vi "SubPanel.vi"(0 "DVR In":refnum<data-value>, 5 "Speed Mode":string, 11 "error in (no error)":errorcluster) -> (4 "DVR Out":refnum<data-value>, 15 "error out":errorcluster)   [LabVIEW 2020, in "Low Speed.lvclass"]
uses:
  Low Speed.lvclass
  Parent/TX Speed.lvclass
  TypeDef/Timing Parameters Cluster.ctl
  TypeDef/User LV2 Mode Select.ctl
  Parent/TypeDefs/TX_Mode Queue Operation Mode.ctl
  TypeDef/Queue Operation Mode.ctl
  <vilib>/Utility/config.llb/Read Key (U32).vi
  I2C Controller Lib.lvlib
  <vilib>/Utility/config.llb/NI_LVConfig.lvlib
panel:
  in  "Time Params":T1={"f_SCL(KHz)"=100, "t_HIGH (ns)"=5000, "t_LOW (ns)"=5000, "t_SU;STA (ns)"=4700, "t_HD;STA (ns)"=4000, "t_SU;DAT (ns)"=2500, "t_HD;DAT (ns)"=2500, "t_SU;STO (ns)"=4000, "t_BUF (ns)"=4700} caption="Time Parameters" {"t_HIGH (ns)" max=1000000 step=1 format="%#.0f"; "t_LOW (ns)" max=1000000 step=1 format="%#.0f"; "f_SCL(KHz)" min=10 max=1000 step=1}
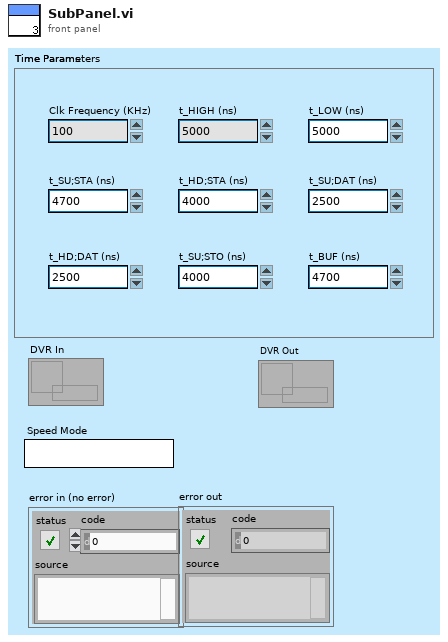
[diagram p1: front panel]
types:
  T1 = typedef "I2C Controller Lib.lvlib/Timing Parameters Cluster.ctl" = cluster{"f_SCL(KHz)":u32, "t_HIGH (ns)":u32, "t_LOW (ns)":u32, "t_SU;STA (ns)":u32, "t_HD;STA (ns)":u32, "t_SU;DAT (ns)":u32, "t_HD;DAT (ns)":u32, "t_SU;STO (ns)":u32, "t_BUF (ns)":u32}
  T2 = cluster{"DVR":refnum<data-value>, "Speed Mode":string, "Time Params":T1, "Event Ref.":refnum<event-registration>}
  T3 = typedef "TX Speed.lvclass/TX_Mode Queue Operation Mode.ctl" = enum16{"Create Q", "Enqueue", "Enqueue N", "Enstack", "Dequeue", "Flush Q", "Close Q"}
  T4 = typedef "I2C Controller Lib.lvlib/User LV2 Mode Select.ctl" = enum16{"Create", "Delete", "Stop"}
  T5 = typedef "I2C Controller Lib.lvlib/Queue Operation Mode.ctl" = enum16{"Create Q", "Enqueue", "Enqueue N", "Enstack", "Dequeue", "Flush Q", "Close Q"}
  T6 = typedef "NI_LVConfig.lvlib/Config Data RefNum.ctl" = refnum<k1>
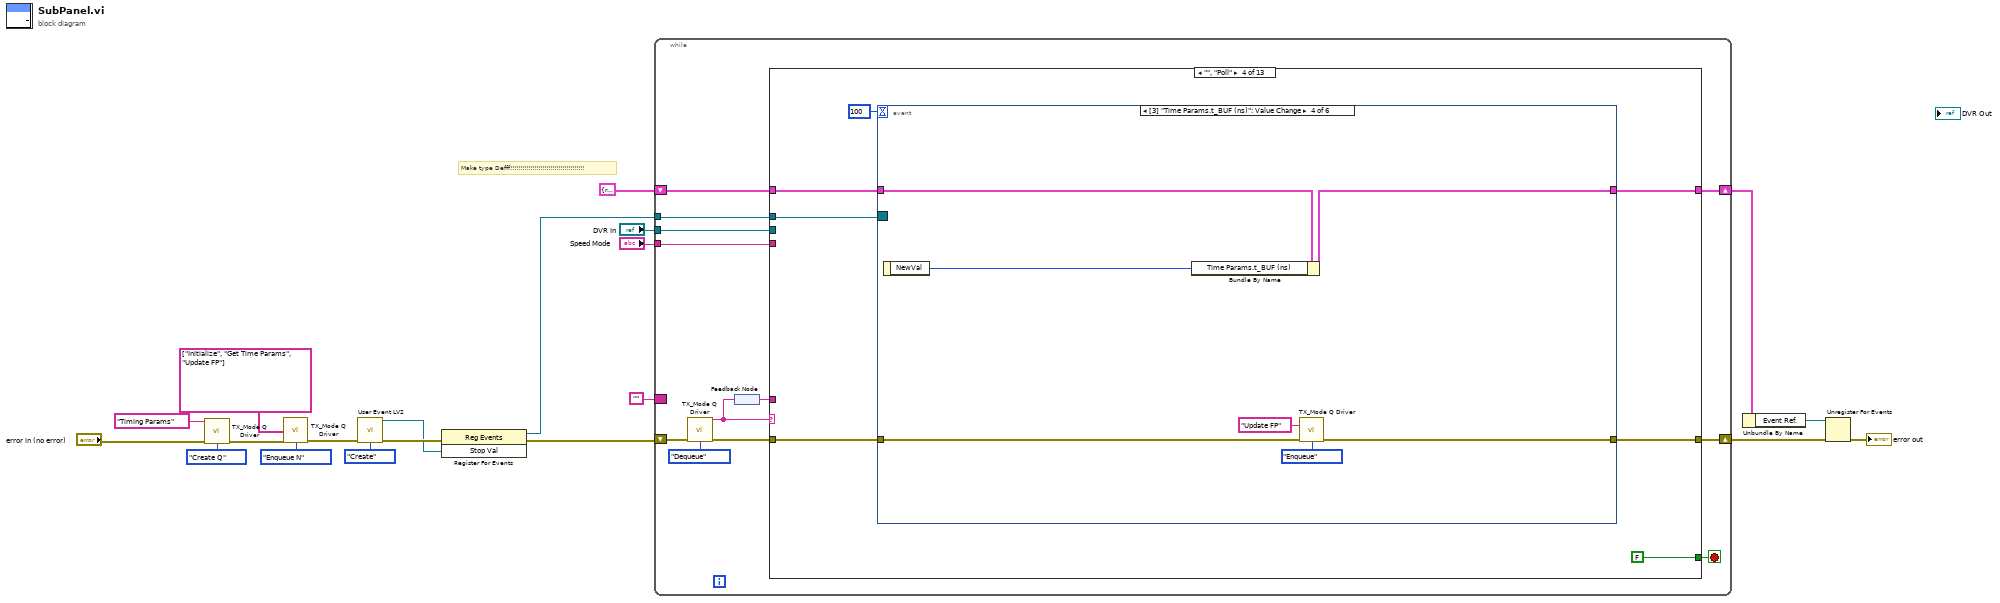
[diagram p0: block diagram]
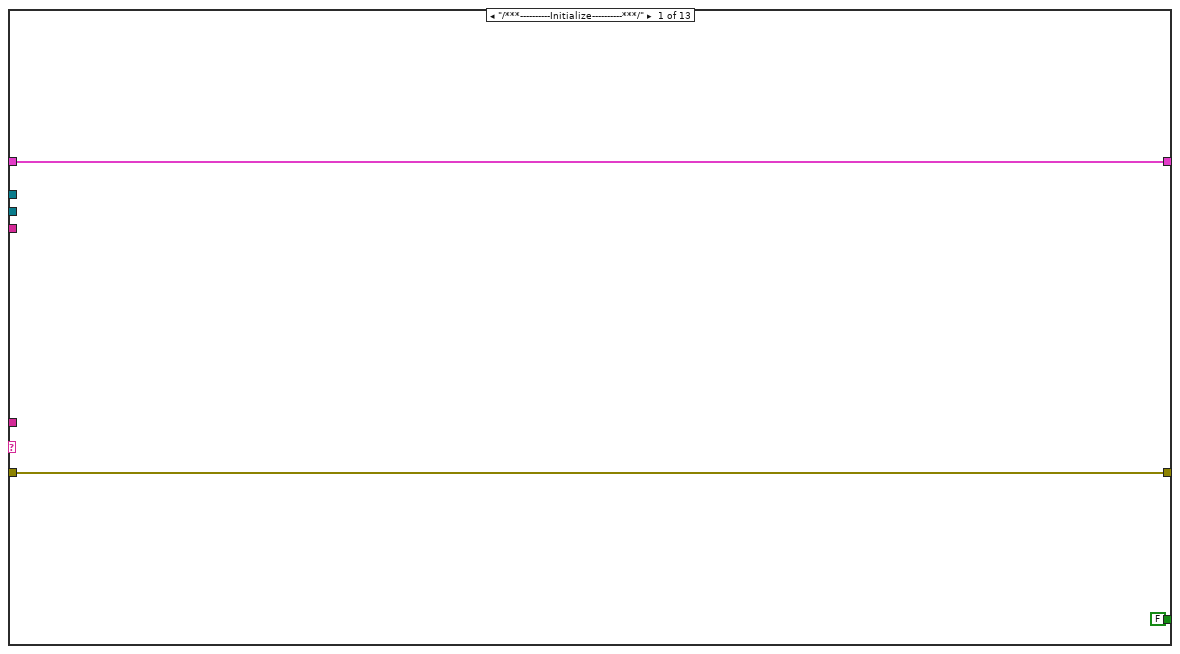
[diagram p2: hidden frame]
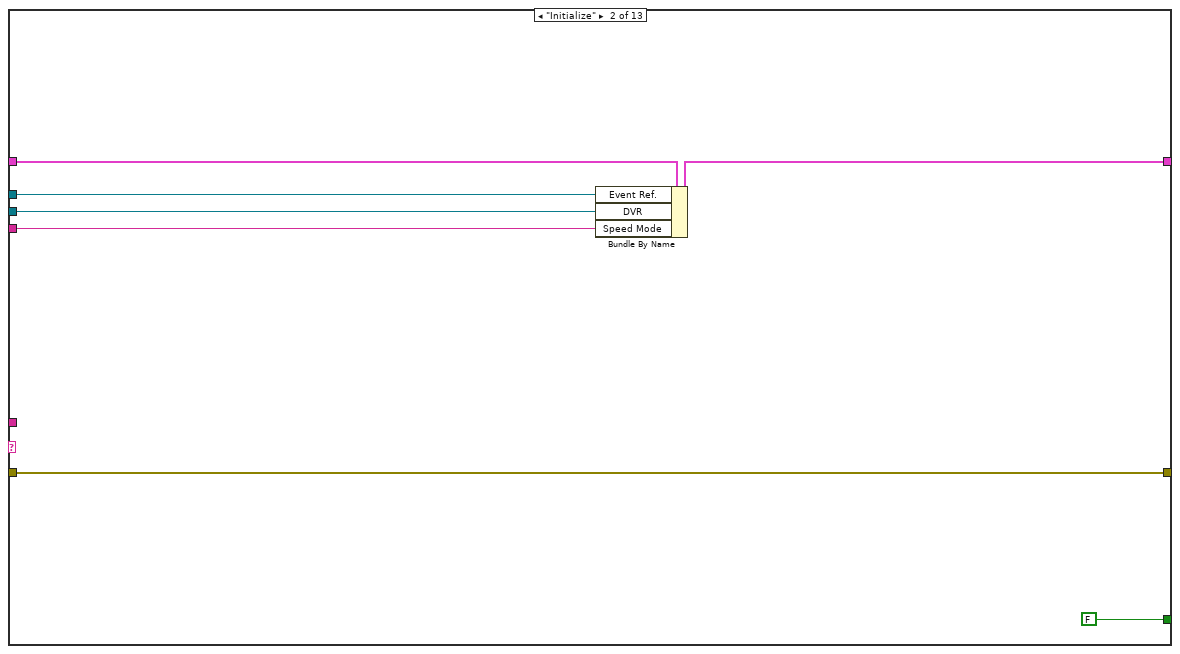
[diagram p3: hidden frame]
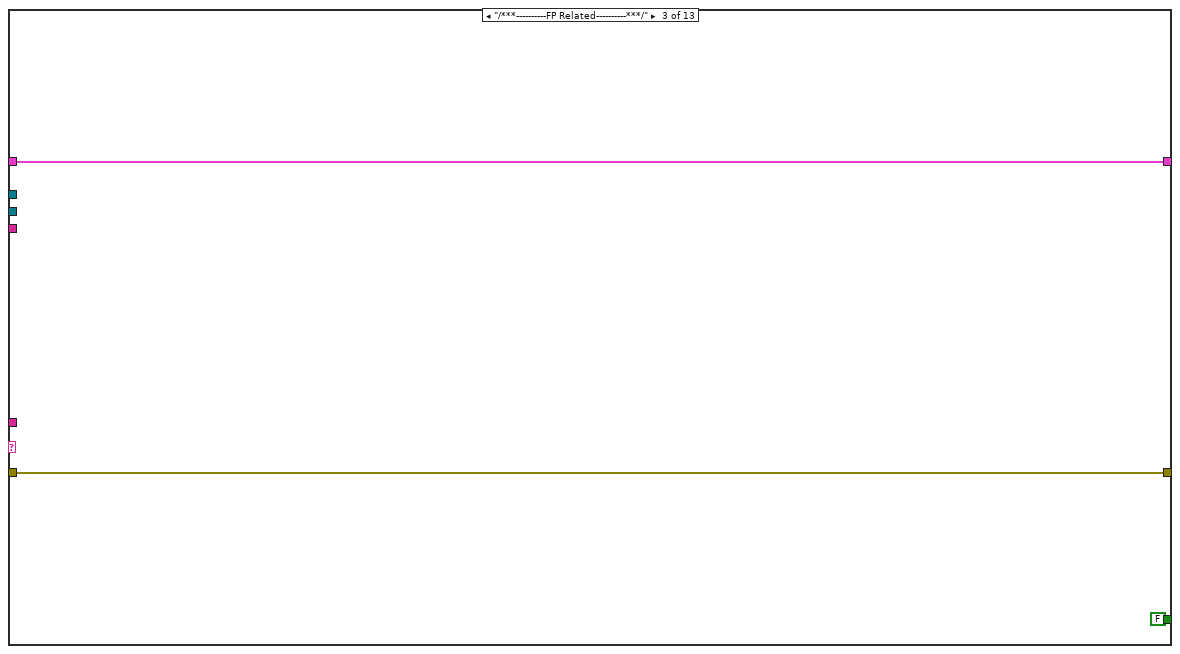
[diagram p4: hidden frame]
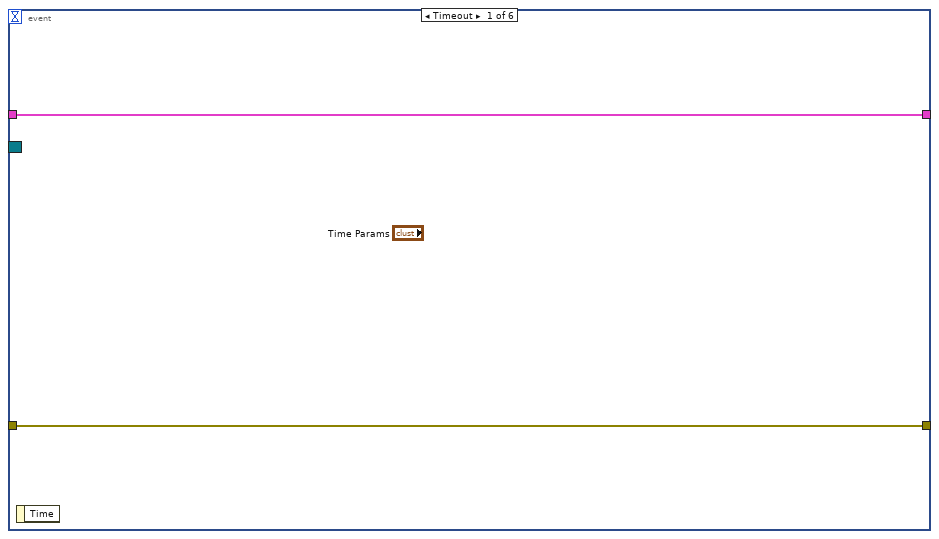
[diagram p5: hidden frame]
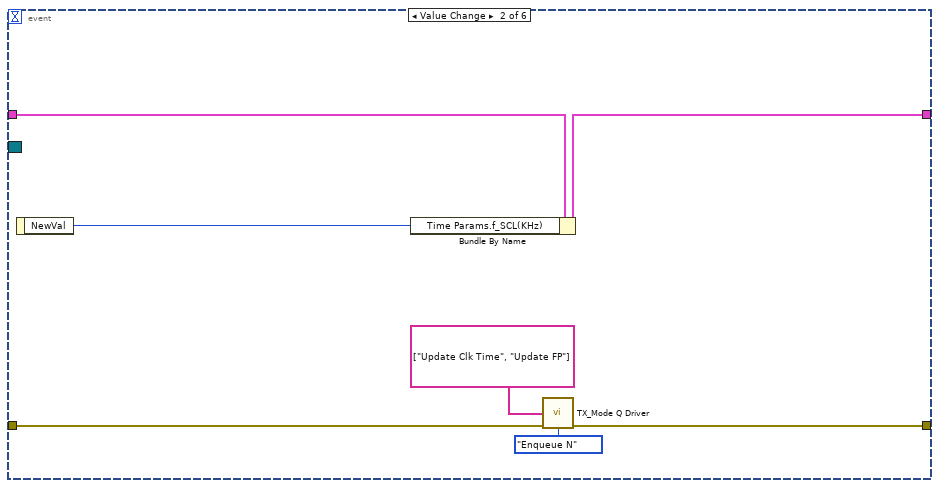
[diagram p6: hidden frame]
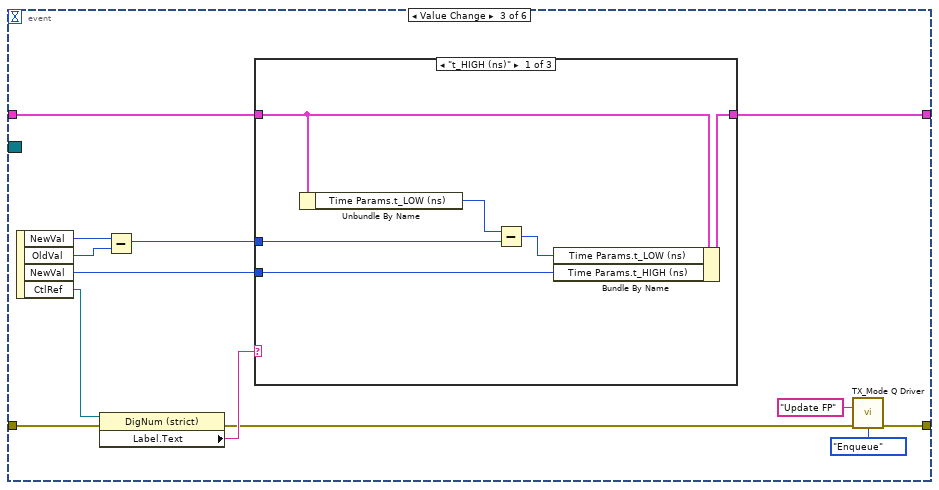
[diagram p7: hidden frame]
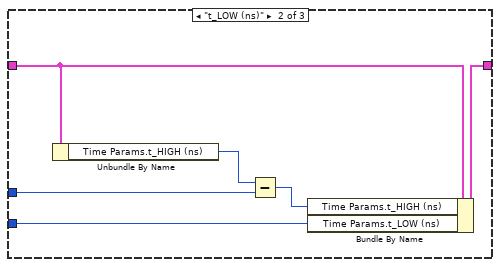
[diagram p8: hidden frame]
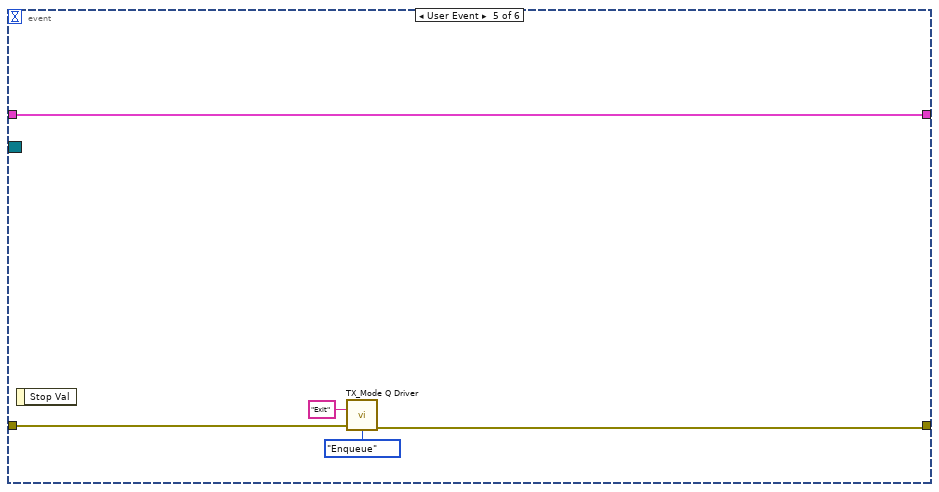
[diagram p10: hidden frame]
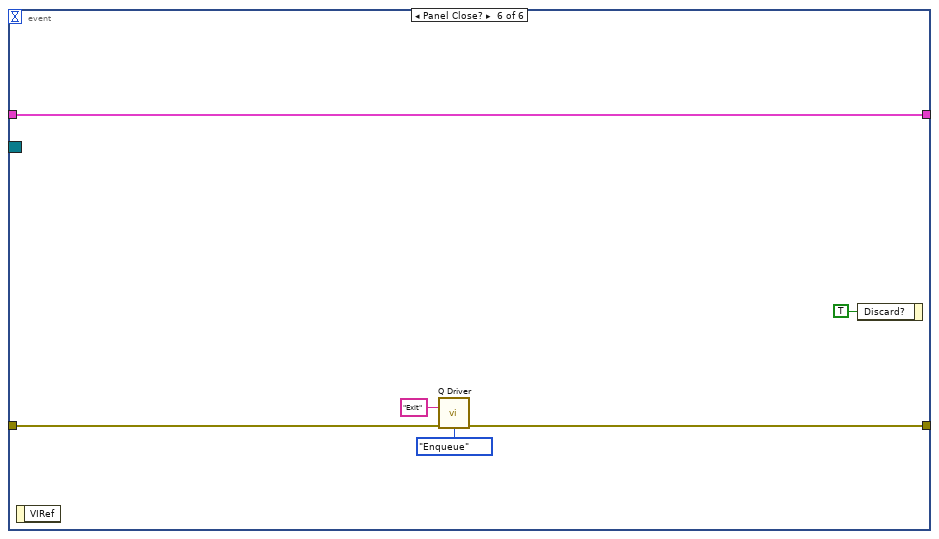
[diagram p11: hidden frame]
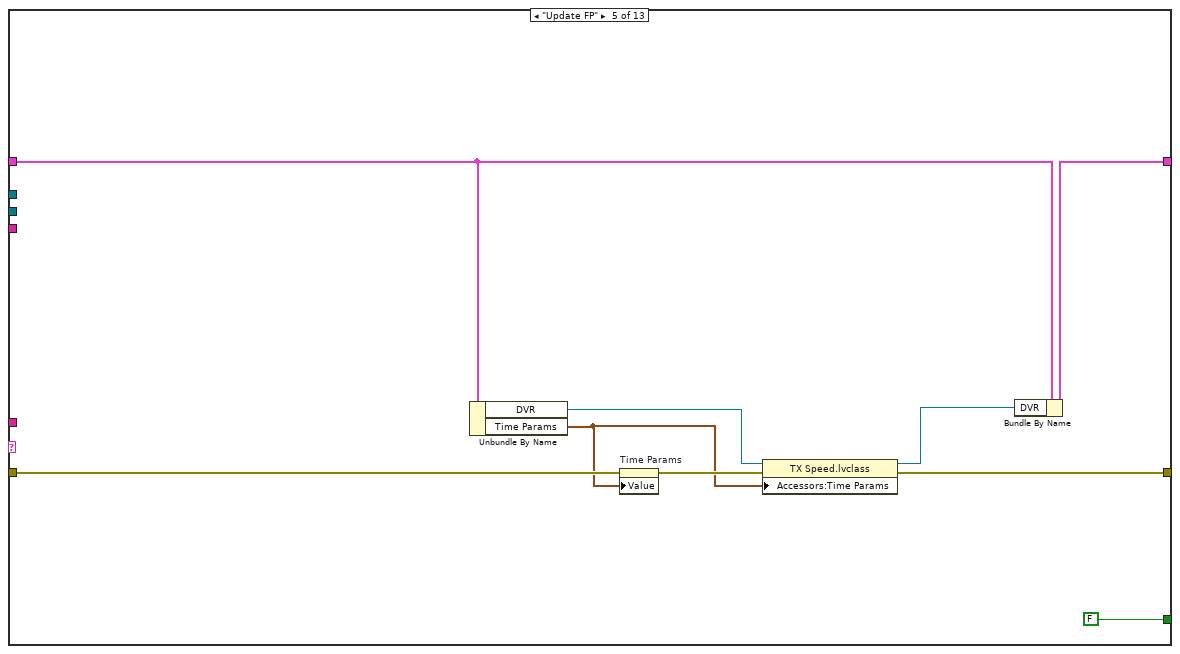
[diagram p12: hidden frame]
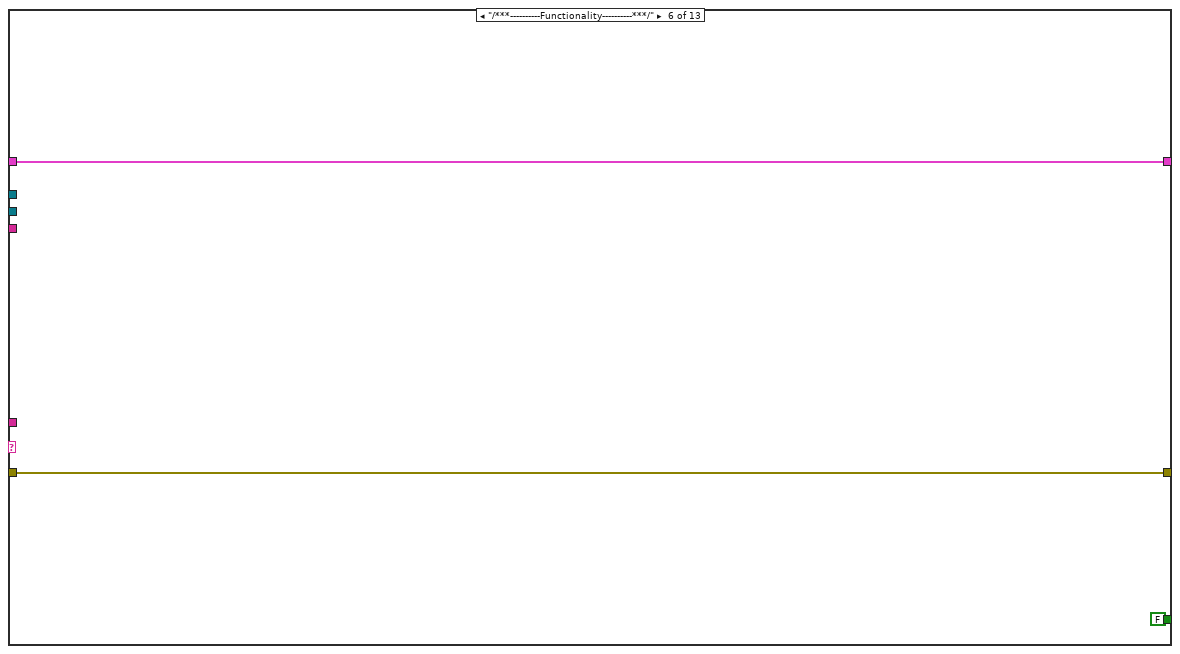
[diagram p13: hidden frame]
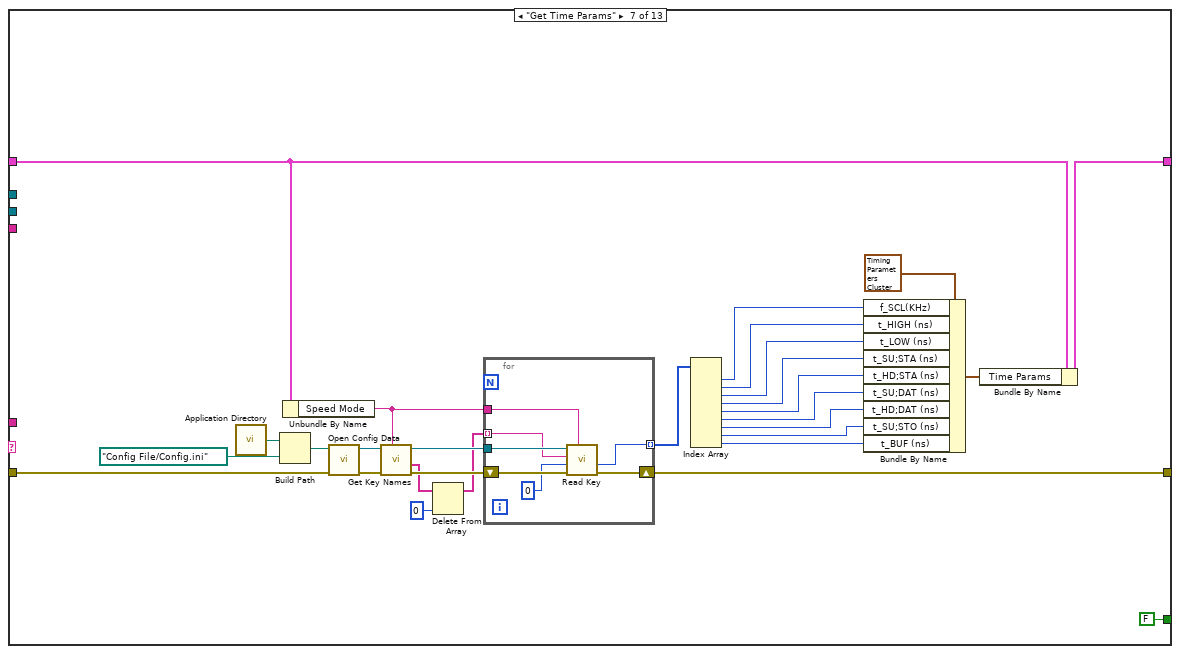
[diagram p14: hidden frame]
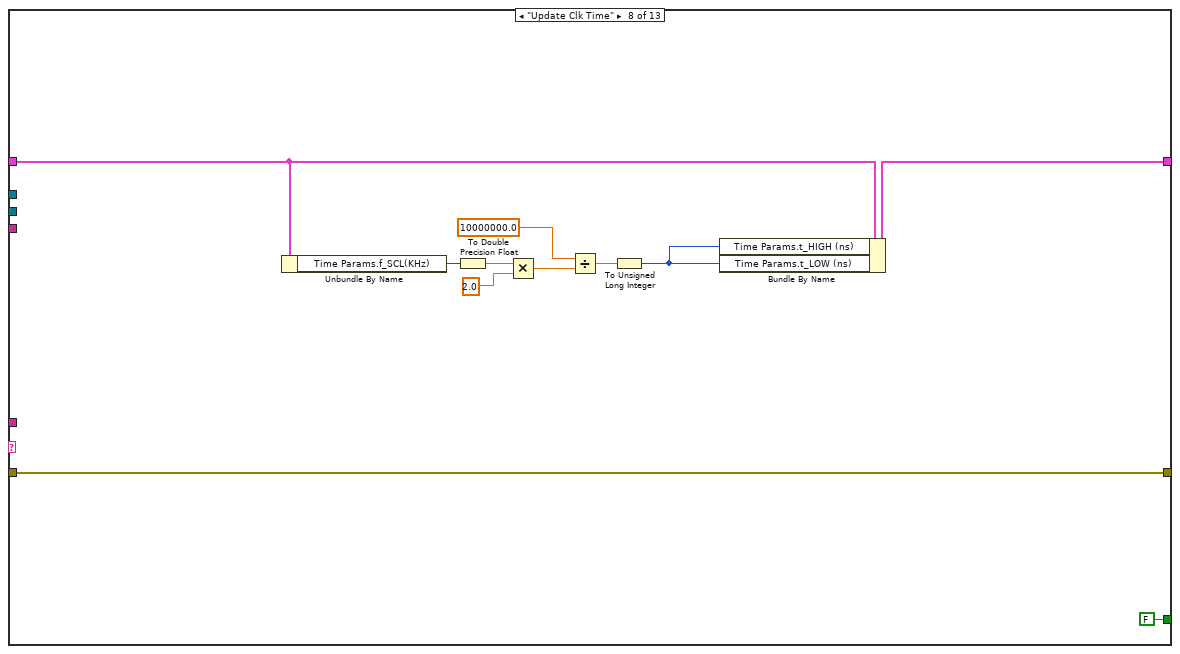
[diagram p15: hidden frame]
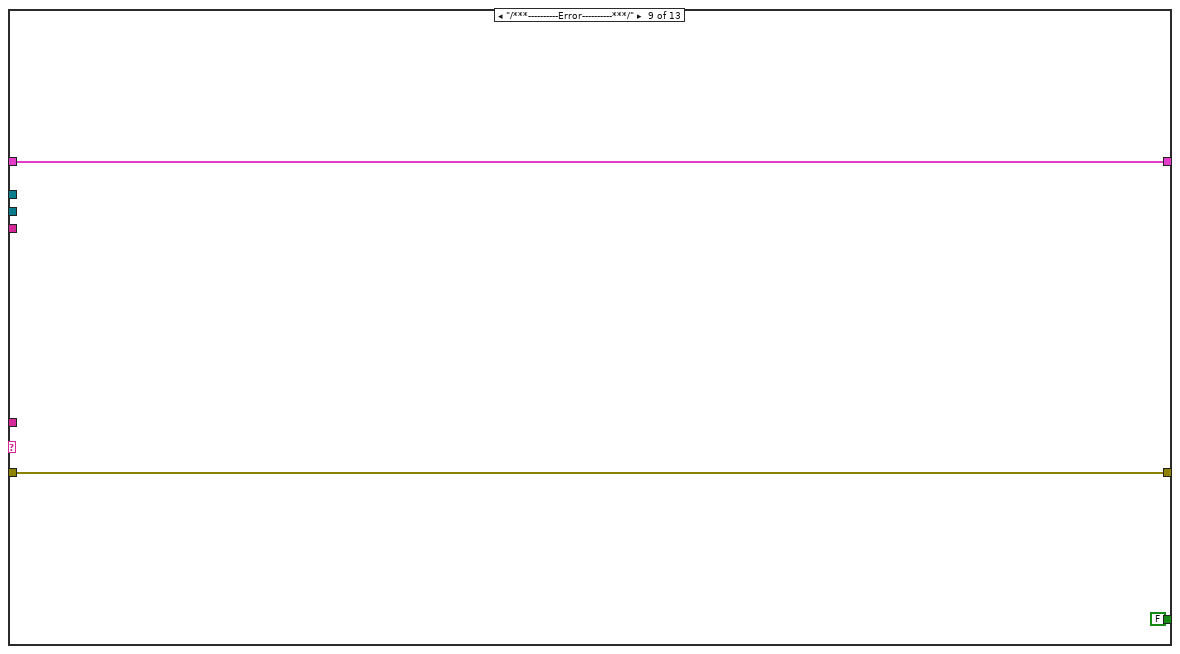
[diagram p16: hidden frame]
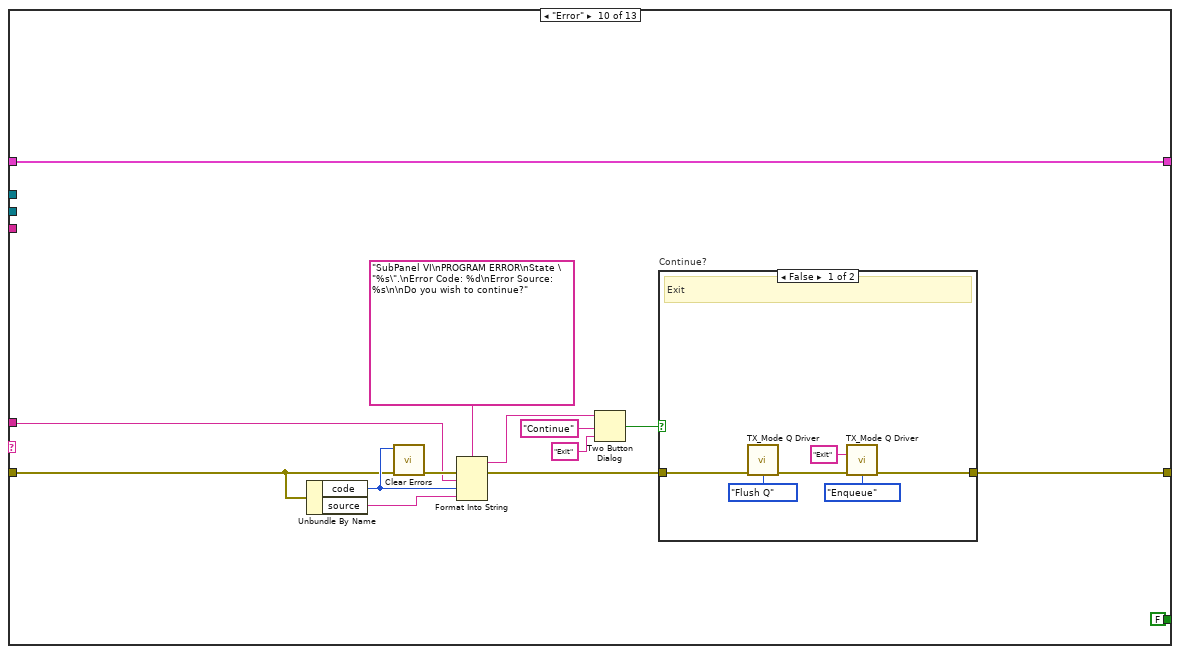
[diagram p17: hidden frame]
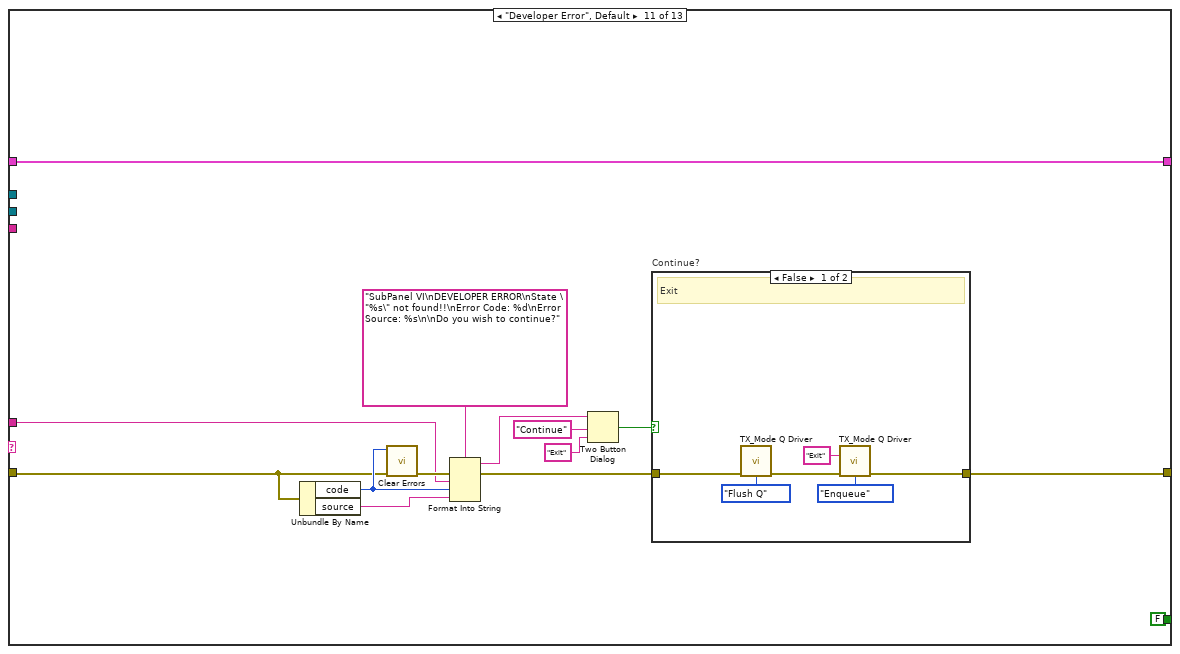
[diagram p19: hidden frame]
diagram:
  # "Make type Defff!!!!!!!!!!!!!!!!!!!!!!!!!!!!!!!!!!!!!"
  n1 = call "TX_Mode Q Driver.vi"("Q Name"="Timing Params", "error in (no error)"="error in (no error)", "Q Operation"=TX_Mode_Queue_Operation_Mode."Create Q") -> ("error out"=w12:errorcluster)  [unwired: 11 in, 1 out]
  n2 = call "TX_Mode Q Driver.vi"("States s[]"=string[] ["Initialize", "Get Time Params", "Update FP"], "error in (no error)"=w12, "Q Operation"=TX_Mode_Queue_Operation_Mode."Enqueue N") -> ("error out"=w8:errorcluster)  [unwired: 11 in, 1 out]
  n3 = call "User Event LV2.vi"("error in (no error)"=w8, "LV2 Mode"=User_LV2_Mode_Select."Create") -> ("Stop Val"=w14:refnum<user-event>, "error out"=w18:errorcluster)  [unwired: 12 in]
  n4 = register-events(error in=w18, w14) -> (reference out=w16:refnum<event-registration>, error out=w17:errorcluster)  [unwired: 1 in]
  n5 = while {
    shift-right: [w32] -> w15
    shift-left: w17 -> [w26]
    shift-right: [w28] -> w4
    shift-left: T2 {"DVR"=refnum, "Speed Mode"="", "Time Params"={"f_SCL(KHz)"=100, "t_HIGH (ns)"=5000, "t_LOW (ns)"=5000, "t_SU;STA (ns)"=4700, "t_HD;STA (ns)"=4000, "t_SU;DAT (ns)"=2500, "t_HD;DAT (ns)"=2500, "t_SU;STO (ns)"=4000, "t_BUF (ns)"=4700}, "Event Ref."=refnum} -> [w29]
    border: "" -> [_]
    tunnel: w16 -> [w31]
    tunnel: "DVR In" -> [w22]
    tunnel: "Speed Mode" -> [w21]
    stop <- w30 stop-if-true
    n6 = call "TX_Mode Q Driver.vi"("error in (no error)"=w26, "Q Operation"=TX_Mode_Queue_Operation_Mode."Dequeue") -> ("State Out"=w24:string, "error out"=w25:errorcluster)  [unwired: 12 in]
    n7 = feedback #1() -> (w23:string)
    n8 = feedback-in #1(w24) -> ()
    n9 = case shown="\"\", \"Poll\"" w24 {
      tunnel: [w35 w42 w45 w52 w110 w117 w145 w163 w166 w169 w191 w211 w214] -> w32
      tunnel: w31 -> [_ w36 _ w50 _ _ _ _ _ _ _ _ _]
      tunnel: [FALSE ("Discard?") FALSE ("Discard?") FALSE ("Discard?") FALSE ("Discard?") FALSE ("Discard?") FALSE ("Discard?") FALSE ("Discard?") FALSE ("Discard?") FALSE ("Discard?") FALSE ("Discard?") FALSE ("Discard?") FALSE ("Discard?") TRUE ("Discard?")] -> w30
      tunnel: w29 -> [w33 w40 w43 w49 w113 w115 w122 w153 w164 w180 w188 w209 w212]
      tunnel: [w33 w39 w43 w48 w107 w115 w119 w162 w164 w180 w188 w209 w212] -> w28
      tunnel: w25 -> [w35 w42 w45 w51 w111 w117 w123 w163 w166 w170 w192 w211 w215]
      tunnel: w23 -> [_ _ _ _ _ _ _ _ _ w168 w190 _ _]
      tunnel: w22 -> [_ w38 _ _ _ _ _ _ _ _ _ _ _]
      tunnel: w21 -> [_ w37 _ _ _ _ _ _ _ _ _ _ _]
      frame "/***----------Initialize----------***/" {
      }
      frame "Initialize" {
        n10 = Bundle By Name(cluster=w40, "Event Ref."=w36, "DVR"=w38, "Speed Mode"=w37) -> (w39:T2)
      }
      frame "/***----------FP Related----------***/" {
      }
      frame "", "Poll" {
        n11 = event shown="[3] \"Time Params.t_BUF (ns)\": Value Change" {
          selector: w50 -> [_ _ _ _ _ _]
          dyn-events: _ -> [_ _ _ _ _ _]
          timeout: 100 -> [_ _ _ _ _ _]
          tunnel: [w54 w59 w63 w88 w95 w100] -> w52
          tunnel: w51 -> [w54 w61 w74 w89 w96 w101]
          tunnel: w49 -> [w53 w60 w73 w94 w99 w105]
          tunnel: [w53 w57 w72 w93 w99 w105] -> w48
          event Timeout {
            n12 = event-data() -> ()  [unwired: 1 in, 1 out]
          }
          event Value Change {
            n13 = event-data() -> ("NewVal"=w55:u32)  [unwired: 1 in]
            n14 = Bundle By Name(cluster=w60, "Time Params.f_SCL(KHz)"=w55) -> (w57:T2)
            n15 = call "TX_Mode Q Driver.vi"("States s[]"=string[] ["Update Clk Time", "Update FP"], "error in (no error)"=w61, "Q Operation"=TX_Mode_Queue_Operation_Mode."Enqueue N") -> ("error out"=w59:errorcluster)  [unwired: 11 in, 1 out]
          }
          event Value Change {
            n16 = event-data() -> ("NewVal"=w67:u32, "OldVal"=w68:u32, "NewVal"=w71:u32, "CtlRef"=w70:refnum<vi>)  [unwired: 1 in]
            n17 = property class="DigNum (strict)"(reference=w70, error in=w74) -> (error out=w64:errorcluster, "Label.Text"=w69:string)  [unwired: 1 out]
            n18 = Subtract(x=w67, y=w68) -> (x-y=w66:u32)
            n19 = case shown="\"t_HIGH (ns)\"" w69 {
              tunnel: w73 -> [w78 w84 w87]
              tunnel: [w80 w86 w87] -> w72
              tunnel: w71 -> [w79 w85 _]
              tunnel: w66 -> [w75 w81 _]
              frame "t_HIGH (ns)" {
                n20 = Unbundle By Name(w78) -> ("Time Params.t_LOW (ns)"=w76:u32)
                n21 = Subtract(x=w76, y=w75) -> (x-y=w77:u32)
                n22 = Bundle By Name(cluster=w78, "Time Params.t_LOW (ns)"=w77, "Time Params.t_HIGH (ns)"=w79) -> (w80:T2)
              }
              frame "t_LOW (ns)" {
                n23 = Unbundle By Name(w84) -> ("Time Params.t_HIGH (ns)"=w82:u32)
                n24 = Subtract(x=w82, y=w81) -> (x-y=w83:u32)
                n25 = Bundle By Name(cluster=w84, "Time Params.t_HIGH (ns)"=w83, "Time Params.t_LOW (ns)"=w85) -> (w86:T2)
              }
              frame Default {
              }
            }
            n26 = call "TX_Mode Q Driver.vi"("State In"="Update FP", "error in (no error)"=w64, "Q Operation"=TX_Mode_Queue_Operation_Mode."Enqueue") -> ("error out"=w63:errorcluster)  [unwired: 11 in, 1 out]
          }
          event Value Change {
            n27 = event-data() -> ("NewVal"=w92:u32)  [unwired: 1 in]
            n28 = Bundle By Name(cluster=w94, "Time Params.t_BUF (ns)"=w92) -> (w93:T2)
            n29 = call "TX_Mode Q Driver.vi"("State In"="Update FP", "error in (no error)"=w89, "Q Operation"=TX_Mode_Queue_Operation_Mode."Enqueue") -> ("error out"=w88:errorcluster)  [unwired: 11 in, 1 out]
          }
          event User Event {
            n30 = event-data() -> ()  [unwired: 1 in, 1 out]
            n31 = call "TX_Mode Q Driver.vi"("State In"="Exit" ("Q Name"), "error in (no error)"=w96, "Q Operation"=TX_Mode_Queue_Operation_Mode."Enqueue") -> ("error out"=w95:errorcluster)  [unwired: 11 in, 1 out]
          }
          event Panel Close? {
            n32 = event-data() -> ()  [unwired: 1 in, 1 out]
            n33 = call "Q Driver.vi"("State In"="Exit" ("Q Name"), "error in (no error)"=w101, "Q Operation"=Queue_Operation_Mode."Enqueue") -> ("error out"=w100:errorcluster)  [unwired: 11 in, 1 out]
            n34 = event-data("Discard?"=TRUE) -> ()  [unwired: 1 in, 1 out]
          }
        }
      }
      frame "Update FP" {
        n35 = Unbundle By Name(w113) -> ("DVR"=w109:refnum<data-value>, "Time Params"=w108:T1)
        n36 = property on="Time Params" class="Clust (strict)"(error in=w111, "Value"=w108) -> (error out=w114:errorcluster)  [unwired: 1 in, 1 out]
        n37 = property class="TX Speed.lvclass"(reference=w109, error in=w114, "Accessors:Time Params"=w108) -> (reference out=w106:refnum<data-value>, error out=w110:errorcluster)
        n38 = Bundle By Name(cluster=w113, "DVR"=w106) -> (w107:T2)
      }
      frame "/***----------Functionality----------***/" {
      }
      frame "Get Time Params" {
        n39 = call <vilib>:"Application Directory.vi"() -> ("Application Directory"=w144:path)
        n40 = Build Path(base path=w144, name or relative path=path "Config File/Config.ini" ("Config.ini")) -> (appended path=w142:path)
        n41 = Unbundle By Name(w122) -> ("Speed Mode"=w121:string)
        n42 = call <vilib>:"Open Config Data.vi"("error in (no error)"=w123, "configuration file path"=w142) -> ("error out"=w141:errorcluster, "refnum"=w127:T6)  [unwired: 7 in, 1 out]
        n43 = call <vilib>:"Get Key Names.vi"("section"=w121, "error in (no error)"=w141, "refnum"=w127) -> ("error out"=w140:errorcluster, "key names"=w126:string[], "refnum out"=w139:T6)  [unwired: 5 in, 1 out]
        n44 = Delete From Array(array=w126, index=0) -> (array with subset deleted=w125:string[])  [unwired: 1 in, 1 out]
        n45 = for {
          shift-right: [w151] -> w145
          shift-left: w140 -> [w152]
          tunnel: w139 -> [w150]
          tunnel: w125 -> [w149] mode=indexing
          tunnel: w121 -> [w148]
          tunnel: [w147] -> w137 mode=indexing
          n46 = call-poly <vilib>:"Read Key.vi"("section"=w148, "error in (no error)"=w152, "default value"=u32 0 ("f_SCL(KHz)"), "key"=w149, "refnum"=w150) -> ("error out"=w151:errorcluster, "value"=w147:u32)  [unwired: 3 in, 2 out]
        }
        n47 = Index Array(array=w137) -> (element #1=w128:u32, element #2=w136:u32, element #3=w135:u32, element #4=w134:u32, element #5=w133:u32, element #6=w132:u32, element #7=w131:u32, element #8=w130:u32, element #9=w129:u32)  [unwired: 9 in]
        n48 = Bundle By Name(cluster=T1 {"f_SCL(KHz)"=100, "t_HIGH (ns)"=5000, "t_LOW (ns)"=5000, "t_SU;STA (ns)"=4700, "t_HD;STA (ns)"=4000, "t_SU;DAT (ns)"=2500, "t_HD;DAT (ns)"=2500, "t_SU;STO (ns)"=4000, "t_BUF (ns)"=4700} ("Time Params"), "f_SCL(KHz)"=w128, "t_HIGH (ns)"=w136, "t_LOW (ns)"=w135, "t_SU;STA (ns)"=w134, "t_HD;STA (ns)"=w133, "t_SU;DAT (ns)"=w132, "t_HD;DAT (ns)"=w131, "t_SU;STO (ns)"=w130, "t_BUF (ns)"=w129) -> (w118:T1)
        n49 = Bundle By Name(cluster=w122, "Time Params"=w118) -> (w119:T2)
      }
      frame "Update Clk Time" {
        n50 = Unbundle By Name(w153) -> ("Time Params.f_SCL(KHz)"=w159:u32)
        n51 = To Double Precision Float(number=w159) -> (double precision float=w158:dbl)
        n52 = Multiply(x=w158, y=2.0) -> (x*y=w155:dbl)
        n53 = Divide(x=10000000.0, y=w155) -> (x/y=w161:dbl)
        n54 = To Unsigned Long Integer(number=w161) -> (unsigned 32bit integer=w160:u32)
        n55 = Bundle By Name(cluster=w153, "Time Params.t_HIGH (ns)"=w160, "Time Params.t_LOW (ns)"=w160) -> (w162:T2)
      }
      frame "/***----------Error----------***/" {
      }
      frame "Error" {
        n56 = Unbundle By Name(w170) -> ("code"=w177:i32, "source"=w176:string)
        n57 = call <vilib>:"Clear Errors.vi"("error in (no error)"=w170, "specific error code to clear (0: all)"=w177) -> ("error out"=w179:errorcluster)  [unwired: 4 in, 1 out]
        n58 = Format Into String(format string="SubPanel VI\nPROGRAM ERROR\nState \"%s\".\nError Code: %d\nError Source: %s\n\nDo you wish to continue?", error in=w179, w168, w177, w176) -> (resulting string=w175:string, error out=w171:errorcluster)  [unwired: 1 in]
        n59 = Two Button Dialog(message=w175, 1:"Exit" ("F button name (\"Cancel\")"), 2:"Continue" ("T button name (\"OK\")")) -> (T button?=w172:bool)
        n60 = case "Continue?" shown="False" w172 {
          tunnel: w171 -> [w186 w187]
          tunnel: [w183 w187] -> w169
          frame False {
            # "Exit"
            n61 = call "TX_Mode Q Driver.vi"("error in (no error)"=w186, "Q Operation"=TX_Mode_Queue_Operation_Mode."Flush Q") -> ("error out"=w184:errorcluster)  [unwired: 12 in, 1 out]
            n62 = call "TX_Mode Q Driver.vi"("State In"="Exit" ("States[]"), "error in (no error)"=w184, "Q Operation"=TX_Mode_Queue_Operation_Mode."Enqueue") -> ("error out"=w183:errorcluster)  [unwired: 11 in, 1 out]
          }
          frame True {
            # "Continue"
          }
        }
      }
      frame "Developer Error", Default {
        n63 = Unbundle By Name(w192) -> ("code"=w199:i32, "source"=w198:string)
        n64 = call <vilib>:"Clear Errors.vi"("error in (no error)"=w192, "specific error code to clear (0: all)"=w199) -> ("error out"=w201:errorcluster)  [unwired: 4 in, 1 out]
        n65 = Format Into String(format string="SubPanel VI\nDEVELOPER ERROR\nState \"%s\" not found!!\nError Code: %d\nError Source: %s\n\nDo you wish to continue?", error in=w201, w190, w199, w198) -> (resulting string=w197:string, error out=w193:errorcluster)  [unwired: 1 in]
        n66 = Two Button Dialog(message=w197, 1:"Exit" ("F button name (\"Cancel\")"), 2:"Continue" ("T button name (\"OK\")")) -> (T button?=w194:bool)
        n67 = case "Continue?" shown="False" w194 {
          tunnel: w193 -> [w207 w208]
          tunnel: [w204 w208] -> w191
          frame False {
            # "Exit"
            n68 = call "TX_Mode Q Driver.vi"("error in (no error)"=w207, "Q Operation"=TX_Mode_Queue_Operation_Mode."Flush Q") -> ("error out"=w205:errorcluster)  [unwired: 12 in, 1 out]
            n69 = call "TX_Mode Q Driver.vi"("State In"="Exit" ("States[]"), "error in (no error)"=w205, "Q Operation"=TX_Mode_Queue_Operation_Mode."Enqueue") -> ("error out"=w204:errorcluster)  [unwired: 11 in, 1 out]
          }
          frame True {
            # "Continue"
          }
        }
      }
      frame "/***----------Exit----------***/" {
      }
      frame "Exit" {
        n70 = call "TX_Mode Q Driver.vi"("error in (no error)"=w215, "Q Operation"=TX_Mode_Queue_Operation_Mode."Flush Q") -> ("error out"=w218:errorcluster)  [unwired: 12 in, 1 out]
        n71 = call "TX_Mode Q Driver.vi"("error in (no error)"=w218, "Q Operation"=TX_Mode_Queue_Operation_Mode."Close Q") -> ("error out"=w214:errorcluster)  [unwired: 12 in, 1 out]
      }
    }
  }
  n72 = Unbundle By Name(w4) -> ("Event Ref."=w3:refnum<event-registration>)
  n73 = Unregister For Events(event registration refnum=w3, error in=w15) -> (error out=→"error out":errorcluster)
